vi "Compute Layout.vi"(0 "State":T1={"Nspeakers"=13, "actions"=[], "Wspeaker"=13, "Wmic"=13, "sel mic"=13, "hover"={"type"=enum."None", "index"=0}, "locked"=FALSE, "states"=[], "sel speak"=13, "selected"=refnum, "Events"={"Mic change"=refnum, "Selection change"=refnum}}, 5 "picture ref":refnum<vi>, 7 "Size":i32) -> (4 "Layout":T6, 6 "Wpict":u32, 8 "Hpict":u32, 10 "Hcontrol":u32)   [LabVIEW 2015, in "HRTF Config.xctl"]
uses:
  HRTF Config.xctl
  Layout.ctl
  Item.ctl
  State.vi
  Hover Data.ctl
  Hover Item.ctl
  Speaker State.ctl
  Events.ctl
  Selection changed.ctl
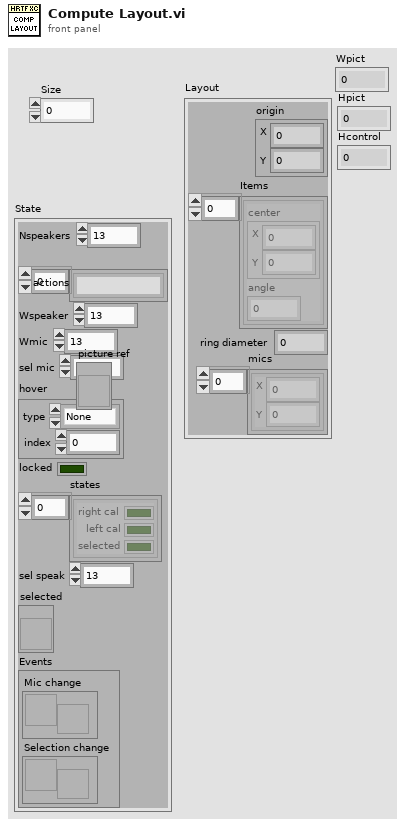
[diagram p1: front panel]
types:
  T1 = typedef "HRTF Config.xctl/State.vi" = cluster{"Nspeakers":i32, "actions":string[], "Wspeaker":i32, "Wmic":i32, "sel mic":i32, "hover":T2, "locked":bool, "states":T4[], "sel speak":i32, "selected":refnum<vi>, "Events":T5}
  T2 = typedef "HRTF Config.xctl/Hover Data.ctl" = cluster{"type":T3, "index":i32}
  T3 = typedef "HRTF Config.xctl/Hover Item.ctl" = enum16{"None", "Speaker", "Mic"}
  T4 = typedef "HRTF Config.xctl/Speaker State.ctl" = cluster{"right cal":bool, "left cal":bool, "selected":bool}
  T5 = typedef "HRTF Config.xctl/Events.ctl" = cluster{"Mic change":refnum<user-event>, "Selection change":refnum<user-event>}
  T6 = typedef "HRTF Config.xctl/Layout.ctl" = cluster{"origin":cluster{"X":i32, "Y":i32}, "Items":T7[], "ring diameter":i32, "mics":cluster{"X":i32, "Y":i32}[]}
  T7 = typedef "HRTF Config.xctl/Item.ctl" = cluster{"center":cluster{"X":i32, "Y":i32}, "angle":dbl}
  T8 = typedef "LVBoundsTypeDef.ctl" = cluster{"Width":u32, "Height":u32}
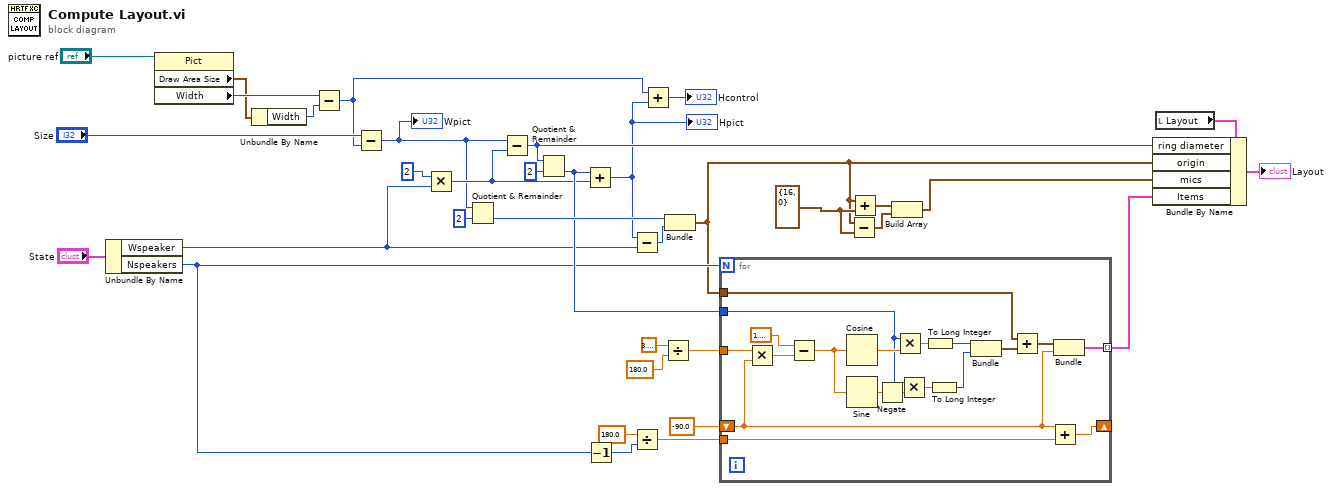
[diagram p0: block diagram]
diagram:
  w21 = cluster{i32, i32} {16, 0} ("output cluster")
  n1 = Unbundle By Name("State") -> ("Wspeaker"=w8:i32, "Nspeakers"=w2:i32)
  n2 = property class="Pict"(reference="picture ref") -> ("Draw Area Size"=w11:T8, "Width"=w12:u32)  [unwired: 1 in, 2 out]
  n3 = Unbundle By Name(w11) -> ("Width"=w13:u32)
  n4 = Subtract(x=w12, y=w13) -> (x-y=w4:u32)
  n5 = Subtract(x="Size", y=w4) -> (x-y=w6:u32)
  "Wpict" <- w6
  n6 = Multiply(x=2 ("y"), y=w8) -> (x*y=w14:i32)
  n7 = Quotient & Remainder(x=w6, y=2) -> (floor(x/y)=w24:u32)  [unwired: 1 out]
  n8 = Subtract(x=w6, y=w14) -> (x-y=w7:u32)
  n9 = Quotient & Remainder(x=w7, y=2) -> (floor(x/y)=w22:u32)  [unwired: 1 out]
  n10 = Add(x=w22, y=w14) -> (x+y=w5:u32)
  "Hpict" <- w5
  n11 = Decrement(x=w2) -> (x-1=w16:i32)
  n12 = Subtract(x=w5, y=w8) -> (x-y=w31:u32)
  n13 = Divide(x=180.0, y=w16) -> (x/y=w29:dbl)
  n14 = Add(x=w4, y=w5) -> (x+y=→"Hcontrol":u32)
  n15 = Divide(x=3.141592653589793, y=180.0) -> (x/y=w26:dbl)
  n16 = Bundle(w24, w31) -> (w1:cluster{u32, u32})  [unwired: 1 in]
  n17 = for {
    N: w2 -> [_]
    tunnel: w1 -> [w40]
    shift-right: [w54] -> _
    shift-left: -90.0 -> [w43]
    tunnel: w29 -> [w53]
    tunnel: w26 -> [w52]
    tunnel: w22 -> [w48]
    tunnel: [w42] -> w25 mode=indexing
    n18 = Multiply(x=w52, y=w43) -> (x*y=w39:dbl)
    n19 = Subtract(x=1.5707963267948966, y=w39) -> (x-y=w38:dbl)
    n20 = Cosine(x=w38) -> (cos(x)=w51:dbl)
    n21 = Sine(x=w38) -> (sin(x)=w47:dbl)
    n22 = Negate(x=w47) -> (-x=w36:dbl)
    n23 = Multiply(x=w48, y=w51) -> (x*y=w50:dbl)
    n24 = Multiply(x=w48, y=w36) -> (x*y=w49:dbl)
    n25 = To Long Integer(number=w50) -> (32bit integer=w46:i32)
    n26 = To Long Integer(number=w49) -> (32bit integer=w45:i32)
    n27 = Bundle(w46, w45) -> (w44:cluster{i32, i32})  [unwired: 1 in]
    n28 = Add(x=w40, y=w44) -> (x+y=w41:cluster{u32, u32})
    n29 = Add(x=w43, y=w53) -> (x+y=w54:dbl)
    n30 = Bundle(w41, w43) -> (w42:cluster{cluster{u32, u32}, dbl})  [unwired: 1 in]
  }
  n31 = Subtract(x=w1, y=w21) -> (x-y=w19:cluster{u32, u32})
  n32 = Add(x=w1, y=w21) -> (x+y=w20:cluster{u32, u32})
  n33 = Build Array(w20, w19) -> (w18:cluster{u32, u32}[])
  n34 = local read "Layout"() -> (w34:T6)
  n35 = Bundle By Name(cluster=w34, "ring diameter"=w7, "origin"=w1, "mics"=w18, "Items"=w25) -> (→"Layout":T6)
